vi "GEMM_CuLab.vi"(7 "Iteration":i32, 11 "Size":i32) -> (3 "Result(s)":dbl format="%.7f")   [LabVIEW 2020]
uses:
  13ac56ee-d342-4fc9-916d-ee8b581d680f.vi
  e733ec95-1f17-4a92-a93c-f13053a3e0ea.vi
  <vilib>/Ngene/CuLab - GPU Accelerated Toolkit/Toolkit/Low_Level/Tensor_Classes/T_Children/T2D/T2D_Children/T2D_SGL/Pull.vi
  <vilib>/Utility/High Resolution Relative Seconds.vi
  <vilib>/Ngene/CuLab - GPU Accelerated Toolkit/Toolkit/Low_Level/GPU_Wrapper/cudart/Memory/PULL/2D/cudart_PULL_Data(SGL_2D).vi
  <vilib>/Ngene/CuLab - GPU Accelerated Toolkit/Toolkit/Low_Level/Tensor_Classes/T_Children/T2D/T2D_Children/T2D_SGL/T2D_SGL.lvclass
  C:/Program Files/National Instruments/LabVIEW 2020/vi.lib/Ngene/CuLab - GPU Accelerated Toolkit/Toolkit/Low_Level/Tensor_Classes/Tensor.lvclass
  C:/Program Files/National Instruments/LabVIEW 2020/vi.lib/Ngene/CuLab - GPU Accelerated Toolkit/Toolkit/Low_Level/Tensor_Classes/T_Children/T2D/T2D.lvclass
  <vilib>/Ngene/CuLab - GPU Accelerated Toolkit/Toolkit/Low_Level/Tensor_Classes/T_Children/T2D/T2D_Children/T2D_SGL/Create.vi
  <vilib>/Ngene/CuLab - GPU Accelerated Toolkit/Toolkit/Low_Level/Tensor_Classes/T_Children/T2D/T2D_Children/T2D_SGL/Push.vi
  <vilib>/Ngene/CuLab - GPU Accelerated Toolkit/Toolkit/API/Linear Algebra/BLAS3/gemm/CU_gemm/CU_Sgemm.vi
  <vilib>/Ngene/CuLab - GPU Accelerated Toolkit/Toolkit/Low_Level/Checkers/Check_Tensor_Ref.vi
  <vilib>/Ngene/CuLab - GPU Accelerated Toolkit/Toolkit/Low_Level/Tensor_Classes/Property/Get_Mem_Desc.vi
  <vilib>/Ngene/CuLab - GPU Accelerated Toolkit/Toolkit/Low_Level/Tensor_Classes/T_Children/T2D/Property/Get_Dims.vi
  <vilib>/Ngene/CuLab - GPU Accelerated Toolkit/Toolkit/Low_Level/GPU_Wrapper/cudart/Memory/Utils/cudart_get_type_size(inBytes).vi
  <vilib>/Ngene/CuLab - GPU Accelerated Toolkit/Toolkit/Low_Level/GPU_Wrapper/cudart/cudart_get_Error_String.vi
  <vilib>/Analysis/NI_AALBase.lvlib
  <vilib>/Ngene/CuLab - GPU Accelerated Toolkit/Toolkit/CuLab.lvlib
panel:
  out "error out":errorcluster
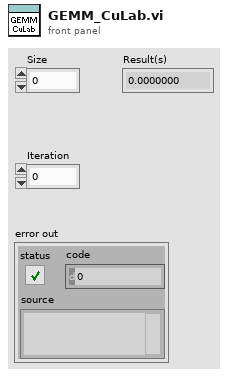
[diagram p1: front panel]
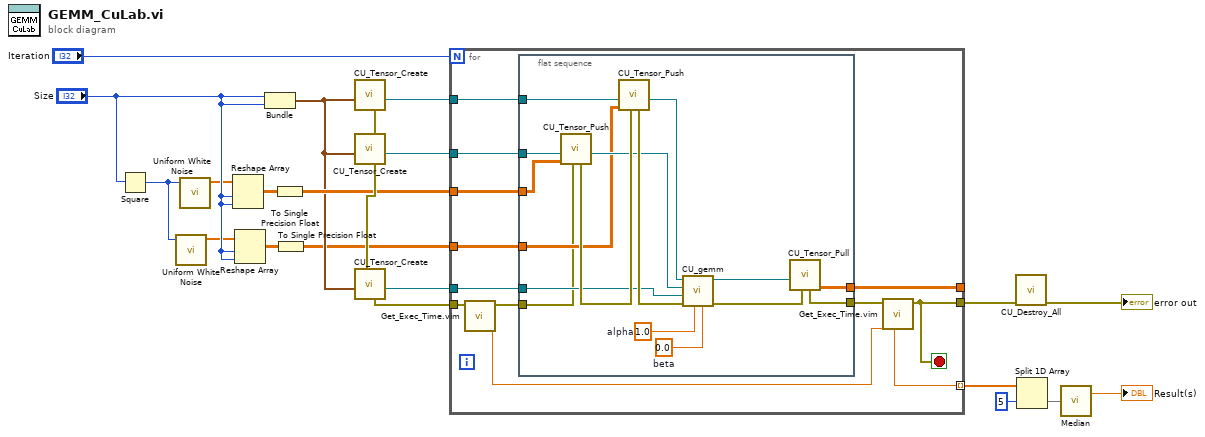
[diagram p0: block diagram]
diagram:
  n1 = Square(x="Size") -> (x^2=w9:i32)
  n2 = call <vilib>:"Uniform White Noise.vi"("samples"=w9) -> ("uniform white noise"=w12:dbl[])  [unwired: 9 in, 1 out]
  n3 = call <vilib>:"Uniform White Noise.vi"("samples"=w9) -> ("uniform white noise"=w13:dbl[])  [unwired: 9 in, 1 out]
  n4 = Reshape Array(w13, "Size", "Size") -> (w10:dbl[][])
  n5 = Reshape Array(w12, "Size", "Size") -> (w11:dbl[][])
  n6 = Bundle("Size"="Size", "Size"="Size") -> (w5:cluster{"Size":i32, "Size":i32})  [unwired: 1 in]
  n7 = To Single Precision Float(number=w10) -> (single precision float=w16:sgl[][])
  n8 = To Single Precision Float(number=w11) -> (single precision float=w4:sgl[][])
  n9 = call-poly <vilib>:"CU_Tensor_Create.vi"("T2D_Dims"=w5) -> ("T2D_SGL out"=w15:refnum<class "T2D_SGL.lvclass">, "error out"=w18:errorcluster)  [unwired: 9 in]
  n10 = call-poly <vilib>:"CU_Tensor_Create.vi"("error in (no error)"=w18, "T2D_Dims"=w5) -> ("T2D_SGL out"=w14:refnum<class "T2D_SGL.lvclass">, "error out"=w17:errorcluster)  [unwired: 8 in]
  n11 = call-poly <vilib>:"CU_Tensor_Create.vi"("error in (no error)"=w17, "T2D_Dims"=w5) -> ("T2D_SGL out"=w8:refnum<class "T2D_SGL.lvclass">, "error out"=w20:errorcluster)  [unwired: 8 in]
  n12 = for {
    N: "Iteration" -> [_]
    tunnel: w16 -> [w31]
    tunnel: w4 -> [w30]
    tunnel: w15 -> [w33]
    tunnel: w14 -> [w34]
    tunnel: w8 -> [w29]
    tunnel: [w32] -> w7
    tunnel: [w25] -> w19 mode=indexing
    tunnel: w20 -> [w24]
    tunnel: [w23] -> _
    stop <- w32 stop-if-true
    n13 = call "Get_Exec_Time.vim"("error in (no error)"=w24) -> ("T(n)"=w26:dbl, "error out"=w28:errorcluster)  [unwired: 6 in, 1 out]
    n14 = flat-sequence {
      tunnel: w34 -> [w47]
      tunnel: w33 -> [w45]
      tunnel: w31 -> [w40]
      tunnel: w30 -> [w39]
      tunnel: w29 -> [w38]
      tunnel: w28 -> [w37]
      tunnel: [w36] -> w27
      tunnel: [w35] -> w23
      frame #0 {
        w49 = sgl 0.0  # beta
        w50 = sgl 1.0  # alpha
        n15 = call-poly <vilib>:"CU_Tensor_Push.vi"("error in (no error)"=w37, "CPU_Data_2D_SGL"=w40, "T2D_SGL in"=w47) -> ("T2D_SGL out"=w41:refnum<class "T2D_SGL.lvclass">, "error out"=w46:errorcluster)  [unwired: 7 in]
        n16 = call-poly <vilib>:"CU_Tensor_Push.vi"("error in (no error)"=w46, "CPU_Data_2D_SGL"=w39, "T2D_SGL in"=w45) -> ("T2D_SGL out"=w42:refnum<class "T2D_SGL.lvclass">, "error out"=w43:errorcluster)  [unwired: 7 in]
        n17 = call-poly <vilib>:"CU_gemm.vi"("beta"=w49, "alpha"=w50, "error in (no error)"=w43, "C"=w38, "B"=w41, "A"=w42) -> ("error out"=w48:errorcluster, "C out"=w44:refnum<class "T2D_SGL.lvclass">)  [unwired: 4 in]
        n18 = call-poly <vilib>:"CU_Tensor_Pull.vi"("error in (no error)"=w48, "T2D_SGL in"=w44) -> ("2D_SGL_Data"=w35:sgl[][], "error out"=w36:errorcluster)  [unwired: 7 in, 1 out]
      }
    }
    n19 = call "Get_Exec_Time.vim"("T(n-1)"=w26, "error in (no error)"=w27) -> ("error out"=w32:errorcluster, "dT"=w25:dbl)  [unwired: 5 in, 1 out]
  }
  n20 = call <vilib>:"CU_Destroy_All.vi"("error in"=w7) -> ("error out"=→"error out":errorcluster)  [unwired: 10 in]
  n21 = Split 1D Array(array=w19, index=5) -> (second subarray=w1:dbl[])  [unwired: 1 out]
  n22 = call <vilib>:"Median.vi"("X"=w1) -> ("median"=→"Result(s)":dbl)  [unwired: 1 out]
